vi "Check Time Out.vi"(8 "error in (no error)":errorcluster, 11 "Timed Door in":refnum<class "Timed Door.lvclass">) -> (0 "error out":errorcluster)   [LabVIEW 2018, in "Timed Door.lvclass"]
uses:
  Timed Door.lvclass
  C:/GitClones/LGP5-Resources/LVOOP/Interfaces/Timed Door/Classes/Door/Door.lvclass
  Timed Door.lvclass/Timed Door.ctl
  Get Alarm DVR.vi
  Get Target Time Elapsed Event.vi
  Get Time Door Has Been Open.vi
  Alarm/Alarm.lvclass
panel:
  out "Open Door Time":dbl
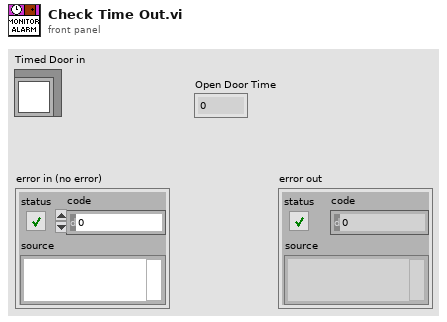
[diagram p1: front panel]
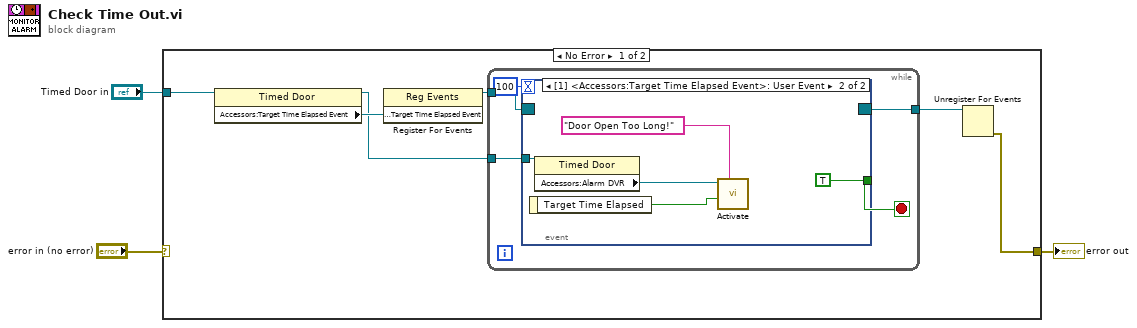
[diagram p0: block diagram]
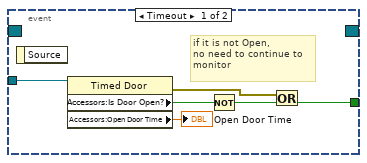
[diagram p2: hidden frame]
diagram:
  n1 = case shown="No Error" "error in (no error)" {
    selector: "error in (no error)" -> [_ w26]
    tunnel: "Timed Door in" -> [w9 _]
    tunnel: [w4 w26] -> w1
    frame No Error {
      n2 = property class="Timed Door"(reference=w9) -> (reference out=w6:refnum<class "Timed Door.lvclass">, "Accessors:Target Time Elapsed Event"=w7:refnum<user-event>)  [unwired: 1 in, 1 out]
      n3 = register-events(w7) -> (reference out=w8:refnum<event-registration>)  [unwired: 2 in, 1 out]
      n4 = while {
        tunnel: w8 -> [w14]
        tunnel: w6 -> [w13]
        tunnel: [w10] -> w5
        stop <- w12 stop-if-true
        n5 = event shown="[1] <Accessors:Target Time Elapsed Event>: User Event" {
          selector: w14 -> [_ _]
          dyn-events: [_ _] -> w10
          timeout: 100 -> [_ _]
          tunnel: w13 -> [w20 w24]
          tunnel: [w16 TRUE] -> w12
          event Timeout {
            # "if it is not Open, \nno need to continue to\nmonitor"
            n6 = event-data() -> ()  [unwired: 1 in, 1 out]
            n7 = property class="Timed Door"(reference=w20) -> (error out=w15:errorcluster, "Accessors:Is Door Open?"=w19:bool, "Accessors:Open Door Time"=→"Open Door Time":dbl)  [unwired: 1 in, 1 out]
            n8 = Not(x=w19) -> (.not. x?=w18:bool)
            n9 = Or(x=w15, y=w18) -> (x .or. y?=w16:bool)
          }
          event User Event {
            n10 = event-data() -> ("Target Time Elapsed"=w21:bool)  [unwired: 1 in]
            n11 = property class="Timed Door"(reference=w24) -> ("Accessors:Alarm DVR"=w23:refnum<data-value>)  [unwired: 1 in, 2 out]
            n12 = call "Activate.vi"("Alarm Reason"="Door Open Too Long!", "Alarm in"=w21, "Data Value Reference in"=w23) -> ()  [unwired: 8 in, 1 out]
          }
        }
      }
      n13 = Unregister For Events(event registration refnum=w5) -> (error out=w4:errorcluster)  [unwired: 1 in]
    }
    frame Error {
    }
  }
  "error out" <- w1
